vi "Load Wavform From TDMS.vi"(0 "TDMS File Path":path, 5 "Waveform Name (File Name)":string, 7 "Normalize Waveform? (T)":bool=TRUE, 11 "error in (no error)":errorcluster) -> (4 "Waveform":T1={"Waveform Name"="Wfm", "Waveform"={"x0"=0.0, "dx"=0.0, "y"=[]}, "Signal Bandwidth (Hz)"=0.0, "PAPR (dB)"=0.0, "Burst Length (s)"=0.0, "Sample Rate"=0.0, "Burst Start Locations"=[], "Burst Stop Locations"=[], "Idle Duration Present?"=FALSE, "Runtime Scaling"=0.0} {"Runtime Scaling" format="%#_6p"; "Sample Rate" format="%#_6p"; "Burst Length (s)" format="%#_6p"; "PAPR (dB)" format="%.2f"; "Signal Bandwidth (Hz)" format="%.2f"; "Waveform"."y" format="%.2f"; "Waveform"."dx" format="%^.2e"; "Waveform"."x0" format="%^.2e"}, 15 "error out":errorcluster)   [LabVIEW 2016, in "SG.lvlib"]
uses:
  SG.lvlib
  Typedefs/Waveform.ctl
  Utilities/RDLUtilities.lvlib
  <instrlib>/niRFSGPlayback/niRFSGPlayback Read Waveform From File (1 Wfm,TDMS, CSG).vi
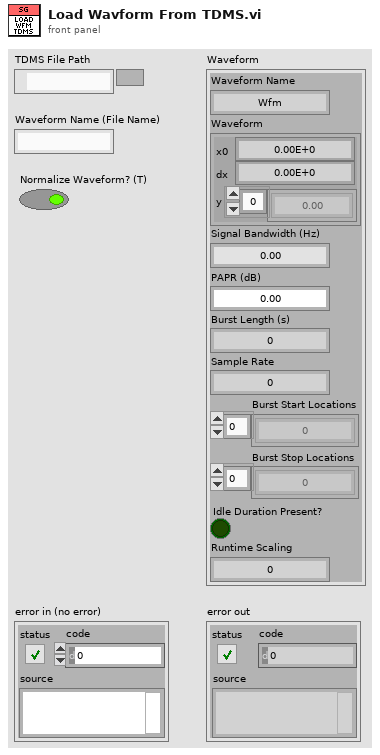
[diagram p1: front panel]
types:
  T1 = typedef "SG.lvlib/Waveform.ctl" = cluster{"Waveform Name":string, "Waveform":cluster{"x0":dbl, "dx":dbl, "y":csg[]}, "Signal Bandwidth (Hz)":dbl, "PAPR (dB)":dbl, "Burst Length (s)":dbl, "Sample Rate":dbl, "Burst Start Locations":i32[], "Burst Stop Locations":i32[], "Idle Duration Present?":bool, "Runtime Scaling":dbl}
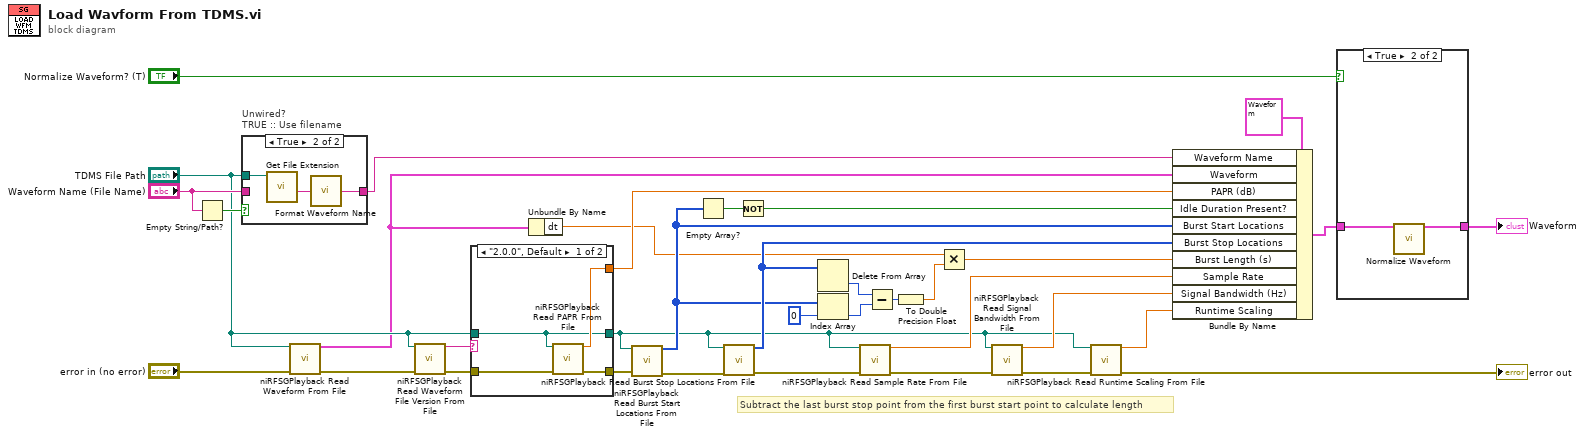
[diagram p0: block diagram]
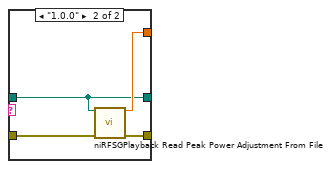
[diagram p2: hidden frame]
diagram:
  # "Subtract the last burst stop point from the first burst start point to calculate length"
  n1 = Empty String/Path?(string/path="Waveform Name (File Name)") -> (empty?=w28:bool)
  n2 = case "Unwired?\nTRUE :: Use filename" shown="True" w28 {
    tunnel: [w36 w37] -> w26
    tunnel: "Waveform Name (File Name)" -> [w36 _]
    tunnel: "TDMS File Path" -> [_ w39]
    frame False {
    }
    frame True {
      n3 = call <vilib>:"Get File Extension.vi"("file"=w39) -> ("filename without extension"=w38:string)  [unwired: 6 in, 4 out]
      n4 = call "Format Waveform Name.vi"("Waveform File Name"=w38) -> ("Waveform Name"=w37:string)
    }
  }
  n5 = call-poly <instrlib>:"niRFSGPlayback Read Waveform From File.vi"("file path"="TDMS File Path", "error in"="error in (no error)") -> ("waveform"=w14:cluster{"t0":dbl, "dt":dbl, "y":csg[]}, "error out"=w34:errorcluster)  [unwired: 12 in]
  n6 = call <instrlib>:"niRFSGPlayback Read Waveform File Version From File.vi"("file path"="TDMS File Path", "error in"=w34) -> ("waveform file version"=w33:string, "error out"=w32:errorcluster)  [unwired: 12 in]
  n7 = case shown="\"2.0.0\", Default" w33 {
    tunnel: w32 -> [w41 w47]
    tunnel: [w40 w44] -> w2
    tunnel: [w43 w46] -> w30
    tunnel: [w42 w45] -> w29
    tunnel: "TDMS File Path" -> [w40 w44]
    frame "2.0.0", Default {
      n8 = call <instrlib>:"niRFSGPlayback Read PAPR From File.vi"("file path"=w40, "error in"=w41) -> ("PAPR"=w43:dbl, "error out"=w42:errorcluster)  [unwired: 12 in]
    }
    frame "1.0.0" {
      n9 = call <instrlib>:"niRFSGPlayback Read Peak Power Adjustment From File.vi"("file path"=w44, "error in"=w47) -> ("peak power adjustment"=w46:dbl, "error out"=w45:errorcluster)  [unwired: 12 in]
    }
  }
  n10 = Unbundle By Name(w14) -> ("dt"=w13:dbl)
  n11 = call <instrlib>:"niRFSGPlayback Read Burst Start Locations From File.vi"("file path"=w2, "error in"=w29) -> ("burst start locations"=w15:i32[], "error out"=w23:errorcluster)  [unwired: 12 in]
  n12 = Empty Array?(array=w15) -> (empty?=w24:bool)
  n13 = call <instrlib>:"niRFSGPlayback Read Burst Stop Locations From File.vi"("file path"=w2, "error in"=w23) -> ("burst stop locations"=w16:i32[], "error out"=w22:errorcluster)  [unwired: 12 in]
  n14 = Not(x=w24) -> (.not. x?=w10:bool)
  n15 = Delete From Array(array=w16) -> (deleted portion=w17:i32)  [unwired: 2 in, 1 out]
  n16 = Index Array(array=w15, index=0) -> (element=w18:i32)
  n17 = call <instrlib>:"niRFSGPlayback Read Sample Rate From File.vi"("file path"=w2, "error in"=w22) -> ("sample rate"=w6:dbl, "error out"=w7:errorcluster)  [unwired: 12 in]
  n18 = Subtract(x=w17, y=w18) -> (x-y=w20:i32)
  n19 = To Double Precision Float(number=w20) -> (double precision float=w21:dbl)
  n20 = Multiply(x=w13, y=w21) -> (x*y=w12:dbl)
  n21 = call <instrlib>:"niRFSGPlayback Read Signal Bandwidth From File.vi"("file path"=w2, "error in"=w7) -> ("signal bandwidth"=w5:dbl, "error out"=w4:errorcluster)  [unwired: 12 in]
  n22 = call <instrlib>:"niRFSGPlayback Read Runtime Scaling From File.vi"("file path"=w2, "error in"=w4) -> ("runtime scaling"=w1:dbl, "error out"=→"error out":errorcluster)  [unwired: 12 in]
  n23 = Bundle By Name(cluster=T1 {"Waveform Name"="Wfm", "Waveform"={"x0"=0.0, "dx"=0.0, "y"=[]}, "Signal Bandwidth (Hz)"=0.0, "PAPR (dB)"=0.0, "Burst Length (s)"=0.0, "Sample Rate"=0.0, "Burst Start Locations"=[], "Burst Stop Locations"=[], "Idle Duration Present?"=FALSE, "Runtime Scaling"=0.0} ("Waveform"), "Waveform Name"=w26, "Waveform"=w14, "PAPR (dB)"=w30, "Idle Duration Present?"=w10, "Burst Start Locations"=w15, "Burst Stop Locations"=w16, "Burst Length (s)"=w12, "Sample Rate"=w6, "Signal Bandwidth (Hz)"=w5, "Runtime Scaling"=w1) -> (w31:T1)
  n24 = case shown="True" "Normalize Waveform? (T)" {
    tunnel: w31 -> [w48 w50]
    tunnel: [w48 w49] -> w9
    frame False {
    }
    frame True {
      n25 = call "Normalize Waveform.vi"("Waveform In"=w50) -> ("Waveform Out"=w49:T1)  [unwired: 14 in]
    }
  }
  "Waveform" <- w9
